vi "dynamic tag creation and mapping.vi"(8 "error in (no error)":errorcluster, 9 "module configurations":refnum<class "TBM module configuration.lvclass">[](array[class]), 10 "modules":refnum<class "TBM module execution interface.lvclass">[](array[class]), 11 "engine configuration in":refnum<class "Simple Sequencer TBM configuration.lvclass">) -> (0 "error out":errorcluster, 1 "module configurations out":refnum<class "TBM module configuration.lvclass">[](array[class]), 2 "modules out":refnum<class "TBM module execution interface.lvclass">[](array[class]), 3 "engine configuration out":refnum<class "Simple Sequencer TBM configuration.lvclass">)   [LabVIEW 2014, in "Simple Sequencer TBM configuration.lvclass"]
doc: "This VI calls the Dynamic Mapping function for each of the modules that are input. Then for each mapping request made by the modules, this VI checks to see if it needs to make a new tag, and then maps the two channels appropriately."
uses:
  <vilib>/NI/TBM Modules/Sequencer/module/configuration/Simple Sequencer TBM configuration.lvclass
  <vilib>/NI/Tag Bus Module Framework/channel/TBM channel.lvclass
  <vilib>/NI/Tag Bus Module Framework/channel/channel classification.ctl
  <vilib>/NI/Tag Bus Module Framework/module configuration/TBM module configuration.lvclass
  <vilib>/NI/Tag Bus Module Framework/runtime/TBM module execution interface.lvclass
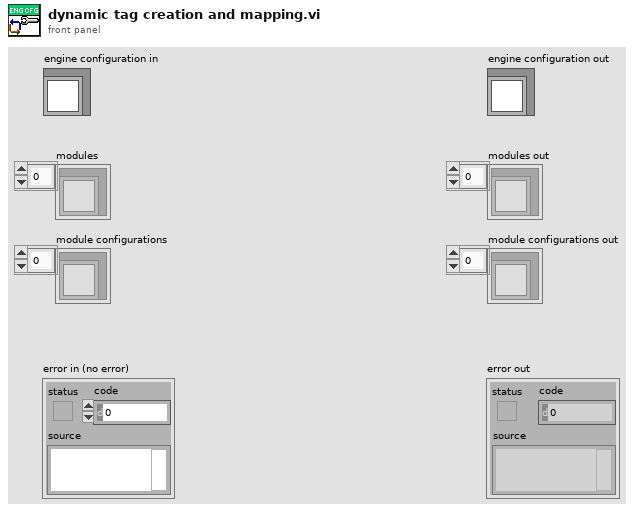
[diagram p1: front panel]
types:
  T1 = typedef "TBM channel.lvclass/channel classification.ctl" = enum16{"input data", "output data", "processing parameter", "processing result"}
  T2 = cluster{"channels":refnum<class "TBM channel.lvclass">[]}
  T3 = typedef "TBM module configuration.lvclass/channel reservation.ctl" = cluster{"local channel":refnum<class "TBM channel.lvclass">, "remote channel":refnum<class "TBM channel.lvclass">}
  T4 = cluster{"channels":refnum<class "TBM channel.lvclass">[]}[]
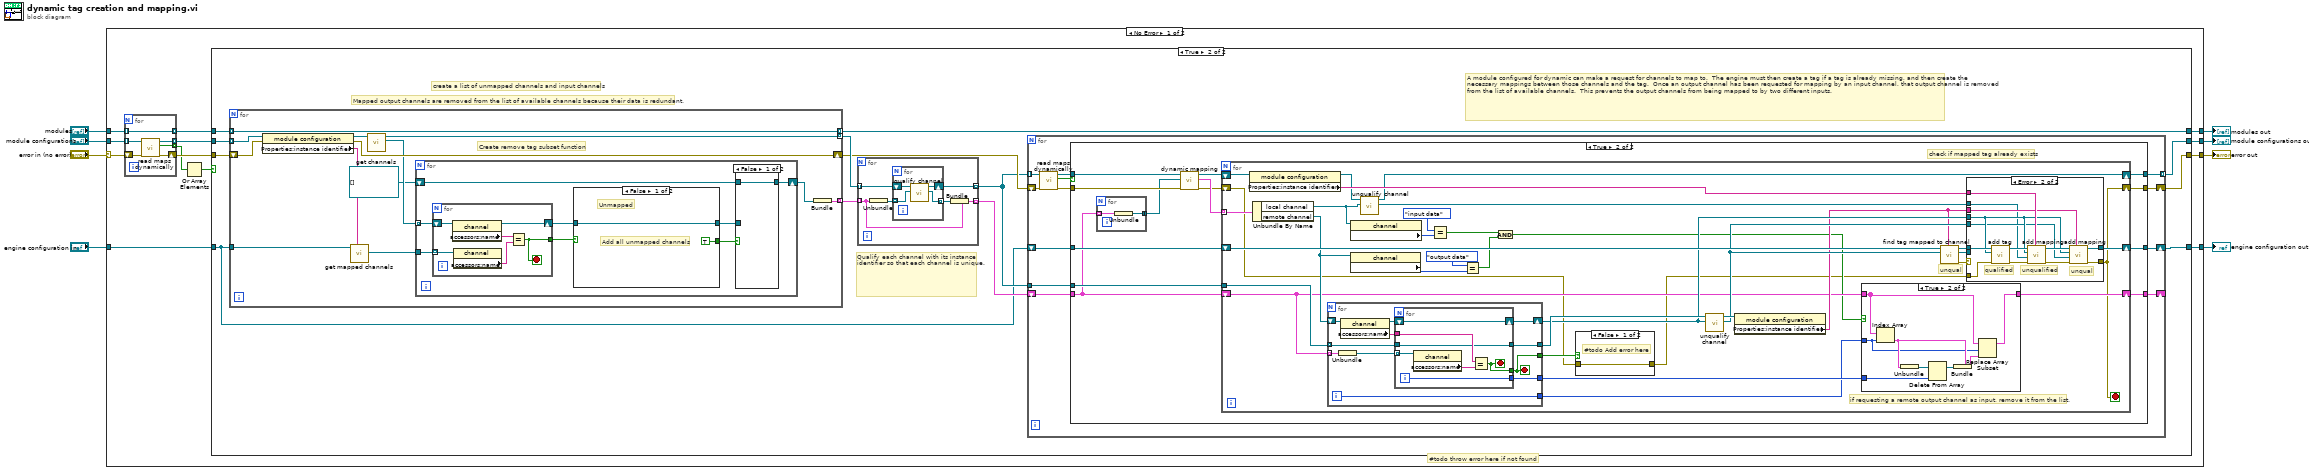
[diagram p0: block diagram]
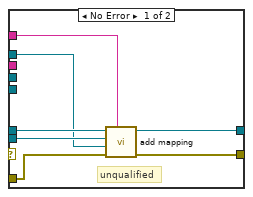
[diagram p6: hidden frame]
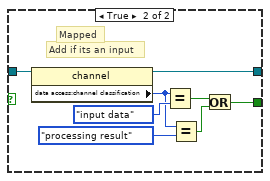
[diagram p7: hidden frame]
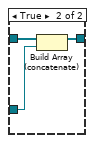
[diagram p8: hidden frame]
diagram:
  n1 = case shown="No Error" "error in (no error)" {
    selector: "error in (no error)" -> [w13 w213]
    tunnel: [w20 w213] -> w7
    tunnel: [w21 w211] -> w6
    tunnel: "engine configuration in" -> [w10 w211]
    tunnel: [w19 w210] -> w4
    tunnel: [w18 w212] -> w3
    tunnel: "module configurations" -> [w15 w212]
    tunnel: "modules" -> [w16 w210]
    frame No Error {
      n2 = for {
        tunnel: [w209] -> w17 mode=indexing
        tunnel: w16 -> [w209] mode=indexing
        tunnel: w15 -> [w208] mode=indexing
        tunnel: [w207] -> w14 mode=indexing
        shift-right: [w205] -> w12
        shift-left: w13 -> [w206]
        tunnel: [w204] -> w11 mode=indexing
        n3 = call-dynamic "read maps dynamically.vi"("error in"=w206, "module configuration in"=w208) -> ("error out"=w205:errorcluster, "maps dynamically"=w204:bool, "module configuration out"=w207:refnum<class "TBM module configuration.lvclass">)  [unwired: 7 in]
      }
      n4 = Or Array Elements(Boolean array=w11) -> (logical OR=w9:bool)
      n5 = case shown="True" w9 {
        tunnel: [w22 w33] -> w21
        tunnel: [w23 w32] -> w20
        tunnel: [w25 w31] -> w19
        tunnel: [w24 w30] -> w18
        tunnel: w17 -> [w25 w29]
        tunnel: w14 -> [w24 w28]
        tunnel: w12 -> [w23 w27]
        tunnel: w10 -> [w22 w26]
        frame False {
        }
        frame True {
          # "A module configured for dynamic can make a request for channels to map to.  The engine must then create a tag if a tag is already missing, and then create the necessary mappings between those channels and the tag.  Once an output channel has been requested for mapping by an input channel, that output channel is removed from the list of available channels.  This prevents the output channels from being mapped to by two different inputs."
          # "Mapped output channels are removed from the list of available channels because their data is redundant."
          # "#todo throw error here if not found"
          # "Qualify each channel with its instance identifier so that each channel is unique."
          # "create a list of unmapped channels and input channels"
          n6 = for {
            tunnel: w28 -> [w164] mode=indexing
            tunnel: w29 -> [w165] mode=indexing
            shift-right: [w170] -> w37
            shift-left: w27 -> [w163]
            tunnel: [w165] -> w31 mode=indexing
            tunnel: w26 -> [w174]
            tunnel: [w171] -> w38 mode=indexing
            tunnel: [w166] -> w36 mode=indexing
            # "Create remove tag subset function"
            n7 = property class="module configuration"(reference=w164, error in=w163) -> (reference out=w173:refnum<class "TBM module configuration.lvclass">, error out=w170:errorcluster, "Properties:instance identifier"=w175:string)
            n8 = call <vilib>:"get mapped channels.vi"("owner"=w175, "engine configuration in"=w174) -> ("channels"=w172:refnum<class "TBM channel.lvclass">[])  [unwired: 8 in, 1 out]
            n9 = call-dynamic "get channels.vi"("module configuration in"=w173) -> ("channels"=w169:refnum<class "TBM channel.lvclass">[], "module configuration out"=w171:refnum<class "TBM module configuration.lvclass">)  [unwired: 9 in]
            n10 = for {
              tunnel: w172 -> [w180]
              tunnel: w169 -> [w181] mode=indexing
              shift-right: [w183] -> w167
              shift-left: refnum<class "TBM channel.lvclass">[] [] ("channels") -> [w182]
              n11 = for {
                tunnel: w180 -> [w198] mode=indexing
                tunnel: [w195] -> w179
                shift-right: [w194] -> w178
                shift-left: w181 -> [w199]
                stop <- w195 stop-if-true
                n12 = property class="channel"(reference=w199) -> (reference out=w194:refnum<class "TBM channel.lvclass">, "accessors:name"=w197:string)  [unwired: 1 in, 1 out]
                n13 = property class="channel"(reference=w198) -> ("accessors:name"=w196:string)  [unwired: 1 in, 2 out]
                n14 = Equal?(x=w197, y=w196) -> (x = y?=w195:bool)
              }
              n15 = case shown="False" w179 {
                tunnel: w178 -> [w185 w189]
                tunnel: [w185 w188] -> w176
                tunnel: [TRUE w187] -> w177
                frame False {
                  # "Add all unmapped channels"
                  # "Unmapped"
                }
                frame True {
                  # "Add if its an input"
                  # "Mapped"
                  n16 = property class="channel"(reference=w189) -> (reference out=w188:refnum<class "TBM channel.lvclass">, "data access:channel classification"=w192:T1)  [unwired: 1 in, 1 out]
                  n17 = Equal?(x=w192, y=channel_classification."input data") -> (x = y?=w191:bool)
                  n18 = Equal?(x=w192, y=channel_classification."processing result") -> (x = y?=w190:bool)
                  n19 = Or(x=w191, y=w190) -> (x .or. y?=w187:bool)
                }
              }
              n20 = case shown="False" w177 {
                tunnel: [w200 w203] -> w183
                tunnel: w182 -> [w200 w202]
                tunnel: w176 -> [_ w201]
                frame False {
                }
                frame True {
                  n21 = Build Array (concatenate)(w202, w201) -> (w203:refnum<class "TBM channel.lvclass">[])
                }
              }
            }
            n22 = Bundle("channels"=w167) -> (w166:T2)  [unwired: 1 in]
          }
          n23 = for {
            tunnel: w38 -> [w158] mode=indexing
            tunnel: w36 -> [w155] mode=indexing
            tunnel: [w153] -> w35 mode=indexing
            tunnel: [w157] -> w34 mode=indexing
            n24 = Unbundle(w155) -> ("channels"=w156:refnum<class "TBM channel.lvclass">[])
            n25 = for {
              tunnel: [w161] -> w154 mode=indexing
              shift-right: [w160] -> w157
              shift-left: w158 -> [w162]
              tunnel: w156 -> [w159] mode=indexing
              n26 = call <vilib>:"qualify channel.vi"("unqualified channel"=w159, "module configuration in"=w162) -> ("qualified channel"=w161:refnum<class "TBM channel.lvclass">, "module configuration out"=w160:refnum<class "TBM module configuration.lvclass">)  [unwired: 8 in]
            }
            n27 = Bundle(cluster=w155, "channels"=w154) -> (w153:T2)
          }
          n28 = for {
            tunnel: w34 -> [w50] mode=indexing
            tunnel: [w44] -> w30 mode=indexing
            shift-right: [w43] -> w32
            shift-left: w37 -> [w48]
            shift-right: [w45] -> w33
            shift-left: w26 -> [w46]
            tunnel: w34 -> [w42]
            shift-right: [w39] -> _
            shift-left: w35 -> [w40]
            n29 = call-dynamic "read maps dynamically.vi"("error in"=w48, "module configuration in"=w50) -> ("error out"=w47:errorcluster, "maps dynamically"=w41:bool, "module configuration out"=w49:refnum<class "TBM module configuration.lvclass">)  [unwired: 7 in]
            n30 = case shown="True" w41 {
              tunnel: w49 -> [w54 w67]
              tunnel: w47 -> [w52 w66]
              tunnel: w46 -> [w53 w64]
              tunnel: [w53 w62] -> w45
              tunnel: [w54 w60] -> w44
              tunnel: [w52 w59] -> w43
              tunnel: w40 -> [w51 w56]
              tunnel: w42 -> [_ w58]
              tunnel: [w51 w57] -> w39
              frame False {
              }
              frame True {
                # "check if mapped tag already exists"
                n31 = for {
                  tunnel: w56 -> [w69] mode=indexing
                  tunnel: [w68] -> w55 mode=concatenating
                  n32 = Unbundle(w69) -> ("channels"=w68:refnum<class "TBM channel.lvclass">[])
                }
                n33 = call-dynamic "dynamic mapping.vi"("error in"=w66, "channels available"=w55, "module configuration in"=w67) -> ("error out"=w63:errorcluster, "reservations"=w65:T3[], "module configuration out"=w61:refnum<class "TBM module configuration.lvclass">)  [unwired: 6 in]
                n34 = for {
                  tunnel: w65 -> [w103] mode=indexing
                  shift-right: [w101] -> w62
                  shift-left: w64 -> [w102]
                  shift-right: [w74] -> w59
                  shift-left: w63 -> [w71]
                  tunnel: w58 -> [w95]
                  shift-right: [w91] -> w60
                  shift-left: w61 -> [w99]
                  shift-right: [w78] -> w57
                  shift-left: w56 -> [w79]
                  stop <- w74 stop-if-true
                  # "if requesting a remote output channel as input, remove it from the list."
                  # "unqual"
                  n35 = property class="module configuration"(reference=w99) -> (reference out=w92:refnum<class "TBM module configuration.lvclass">, "Properties:instance identifier"=w100:string)  [unwired: 1 in, 1 out]
                  n36 = Unbundle By Name(w103) -> ("local channel"=w73:refnum<class "TBM channel.lvclass">, "remote channel"=w86:refnum<class "TBM channel.lvclass">)
                  n37 = for {
                    tunnel: w95 -> [w121] mode=indexing
                    tunnel: w79 -> [w117] mode=indexing
                    tunnel: [w120] -> w94
                    tunnel: [w119] -> w75
                    tunnel: [w118] -> w76
                    shift-right: [w122] -> w88
                    shift-left: w86 -> [w125]
                    tunnel: [w115] -> w72
                    i -> [w119]
                    stop <- w115 stop-if-true
                    n38 = Unbundle(w117) -> ("channels"=w116:refnum<class "TBM channel.lvclass">[])
                    n39 = property class="channel"(reference=w125) -> (reference out=w123:refnum<class "TBM channel.lvclass">, "accessors:name"=w124:string)  [unwired: 1 in, 1 out]
                    n40 = for {
                      tunnel: w116 -> [w132] mode=indexing
                      tunnel: w124 -> [w129]
                      tunnel: [w128] -> w115
                      tunnel: w121 -> [w127]
                      tunnel: [w127] -> w120
                      tunnel: [w126] -> w118
                      shift-right: [w131] -> w122
                      shift-left: w123 -> [w131]
                      i -> [w126]
                      stop <- w128 stop-if-true
                      n41 = property class="channel"(reference=w132) -> ("accessors:name"=w130:string)  [unwired: 1 in, 2 out]
                      n42 = Equal?(x=w129, y=w130) -> (x = y?=w128:bool)
                    }
                  }
                  n43 = property class="channel"(reference=w86) -> ("data access:channel classification"=w83:T1)  [unwired: 1 in, 2 out]
                  n44 = property class="channel"(reference=w73) -> ("data access:channel classification"=w85:T1)  [unwired: 1 in, 2 out]
                  n45 = call <vilib>:"unqualify channel.vi"("qualified channel"=w73, "module configuration in"=w92) -> ("unqualified channel"=w90:refnum<class "TBM channel.lvclass">, "module configuration out"=w91:refnum<class "TBM module configuration.lvclass">)  [unwired: 8 in]
                  n46 = Equal?(x=channel_classification."input data", y=w85) -> (x = y?=w81:bool)
                  n47 = Equal?(x=channel_classification."output data", y=w83) -> (x = y?=w80:bool)
                  n48 = And(x=w81, y=w80) -> (x .and. y?=w77:bool)
                  n49 = case shown="False" w72 {
                    tunnel: w71 -> [w104 w105]
                    tunnel: [w104 w105] -> w70
                    frame False {
                      # "#todo Add error here"
                    }
                    frame True {
                    }
                  }
                  n50 = call <vilib>:"unqualify channel.vi"("qualified channel"=w88, "module configuration in"=w94) -> ("unqualified channel"=w89:refnum<class "TBM channel.lvclass">, "module configuration out"=w93:refnum<class "TBM module configuration.lvclass">)  [unwired: 8 in]
                  n51 = property class="module configuration"(reference=w93) -> ("Properties:instance identifier"=w87:string)  [unwired: 1 in, 2 out]
                  n52 = case shown="True" w77 {
                    tunnel: w79 -> [w106 w110]
                    tunnel: [w106 w107] -> w78
                    tunnel: w76 -> [_ w113]
                    tunnel: w75 -> [_ w108]
                    frame False {
                    }
                    frame True {
                      n53 = Index Array(array=w110, index=w108) -> (element=w111:T2)
                      n54 = Unbundle(w111) -> ("channels"=w114:refnum<class "TBM channel.lvclass">[])
                      n55 = Delete From Array(array=w114, index=w113) -> (array with subset deleted=w112:refnum<class "TBM channel.lvclass">[])  [unwired: 1 in, 1 out]
                      n56 = Bundle(cluster=w111, "channels"=w112) -> (w109:T2)
                      n57 = Replace Array Subset(array=w110, new element=w109, index=w108) -> (w107:T4)
                    }
                  }
                  n58 = call <vilib>:"find tag mapped to channel.vi"("owner"=w87, "channel"=w89, "engine configuration in"=w102) -> ("error out"=w98:errorcluster, "tag"=w96:refnum<class "tag descriptor.lvclass">, "engine configuration out"=w97:refnum<class "Simple Sequencer TBM configuration.lvclass">)  [unwired: 6 in]
                  n59 = case shown="Error" w98 {
                    tunnel: w97 -> [w138 w150]
                    tunnel: w70 -> [w136 w149]
                    tunnel: w96 -> [w139 _]
                    tunnel: w90 -> [w133 w140]
                    tunnel: [w137 w144] -> w101
                    tunnel: [w135 w145] -> w74
                    tunnel: w100 -> [w134 w148]
                    tunnel: w88 -> [_ w142]
                    tunnel: w89 -> [_ w141]
                    tunnel: w87 -> [_ w143]
                    frame No Error {
                      # "unqualified"
                      n60 = call <vilib>:"add mapping.vi"("owner ID"=w134, "error in"=w136, "channel"=w133, "tag descriptor"=w139, "engine configuration"=w138) -> ("error out"=w135:errorcluster, "engine configuration out"=w137:refnum<class "Simple Sequencer TBM configuration.lvclass">)  [unwired: 5 in]
                    }
                    frame Error {
                      # "unqual"
                      # "unqualified"
                      # "qualified"
                      n61 = call <vilib>:"add tag.vi"("error in"=w149, "tag descriptor"=w142, "engine configuration in"=w150) -> ("error out"=w151:errorcluster, "engine configuration out"=w152:refnum<class "Simple Sequencer TBM configuration.lvclass">)  [unwired: 7 in]
                      n62 = call <vilib>:"add mapping.vi"("owner ID"=w148, "error in"=w151, "channel"=w140, "tag descriptor"=w142, "engine configuration"=w152) -> ("error out"=w146:errorcluster, "engine configuration out"=w147:refnum<class "Simple Sequencer TBM configuration.lvclass">)  [unwired: 5 in]
                      n63 = call <vilib>:"add mapping.vi"("owner ID"=w143, "error in"=w146, "channel"=w141, "tag descriptor"=w142, "engine configuration"=w147) -> ("error out"=w145:errorcluster, "engine configuration out"=w144:refnum<class "Simple Sequencer TBM configuration.lvclass">)  [unwired: 5 in]
                    }
                  }
                }
              }
            }
          }
        }
      }
    }
    frame Error {
    }
  }
  "error out" <- w7
  "engine configuration out" <- w6
  "module configurations out" <- w3
  "modules out" <- w4
